vi "DSF.Engine.Memory.Index FIFO.Create.vi"(8 "error in (no error)":errorcluster, 11 "size":u32) -> (0 "error out":errorcluster, 3 "Index FIFO out":refnum<class "DSF.Engine.Memory.Index FIFO.lvclass">)   [LabVIEW 2016, in "DSF.Engine.lvlib" / "DSF.Engine.Memory.Index FIFO.lvclass"]
uses:
  DSF.Engine.Memory.Index FIFO.lvclass
  DSF.Engine.Memory.Index FIFO.lvclass/DSF.Engine.Memory.Index FIFO.ctl
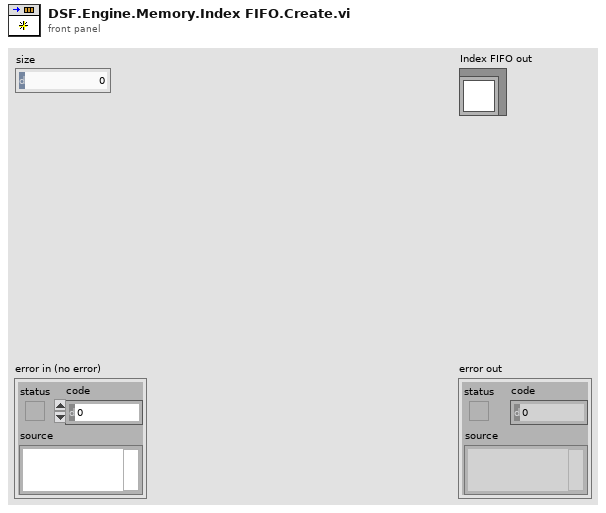
[diagram p1: front panel]
types:
  T1 = cluster{"read mode":enum16{"polling", "blocking"}, "write mode":enum16{"polling", "blocking"}}
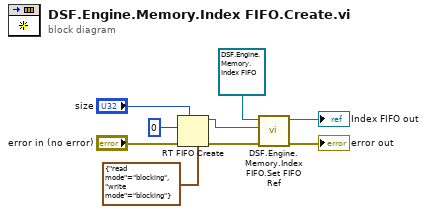
[diagram p0: block diagram]
diagram:
  n1 = RT FIFO Create(1:0, 3:"error in (no error)", 4:"size", 7:T1 {"read mode"=enum."blocking", "write mode"=enum."blocking"} ("r/w modes (polling,polling)")) -> (8:w4:refnum<k33>, 11:w6:errorcluster)  [unwired: 4 in, 1 out]
  n2 = call "DSF.Engine.Memory.Index FIFO.Set FIFO Ref.vi"("error in (no error)"=w6, "FIFO"=w4, "Index FIFO in"=refnum<class "DSF.Engine.Memory.Index FIFO.lvclass"> refnum) -> ("error out"=→"error out":errorcluster, "Index FIFO out"=→"Index FIFO out":refnum<class "DSF.Engine.Memory.Index FIFO.lvclass">)  [unwired: 7 in]
